vi "GLOBAL Time-critical.vi"() -> ()   [LabVIEW 2018]
uses:
  Type Defs/Physical Camera Assignment.ctl
  Type Defs/Camera Type.ctl
panel:
  in  "Live Frame":u16[][][](array[numeric])
  in  "Trigger Ready":bool
  in  "Abort Stage Motion":bool
  in  "Camera Model":string
  in  "Saving Frame":i32
  in  "Active Cameras":T1[](array[typedef])
  in  "Total Frames":i32
  in  "Current Frame":i32
  in  "Streaming":bool
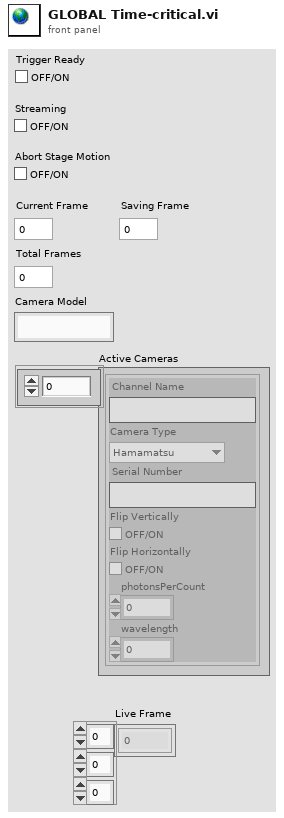
[diagram p1: front panel]
types:
  T1 = typedef "Physical Camera Assignment.ctl" = cluster{"Channel Name":string, "Camera Type":T2, "Serial Number":string, "Flip Vertically":bool, "Flip Horizontally":bool, "photonsPerCount":dbl, "wavelength":i16}
  T2 = typedef "Camera Type.ctl" = enum16{"Hamamatsu"}
diagram:
